vi "Open PNG and convert to 18bit.vi"(8 "error in":errorcluster, 10 "image data":T1={"image type"=0, "image depth"=24, "image"=array[230400 elements], "mask"=[], "colors"=[], "Rectangle"={"left"=0, "top"=0, "right"=320, "bottom"=240}}, 11 "file path (use dialog)":path=path "\\\\vmware-host\\Shared Folders/Downloads/pug.bin") -> (0 "error out":errorcluster, 3 "data":u16[](array[numeric]) format="%.0x")   [LabVIEW 2019]
uses:
  <vilib>/picture/picture.llb/imagedata.ctl
  <userlib>/_OpenG.lib/file/file.llb/File Exists - Scalar__ogtk.vi
panel:
  out "new picture":picture
  out "exists":bool
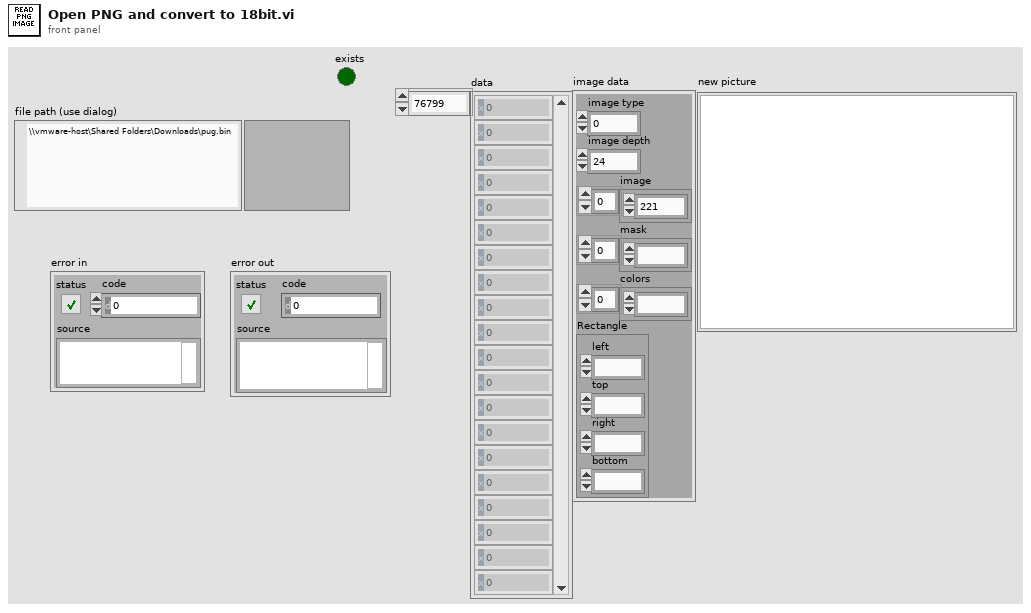
[diagram p1: front panel]
types:
  T1 = typedef "imagedata.ctl" = cluster{"image type":i32, "image depth":i32, "image":u8[], "mask":u8[], "colors":u32[], "Rectangle":cluster{"left":i16, "top":i16, "right":i16, "bottom":i16}}
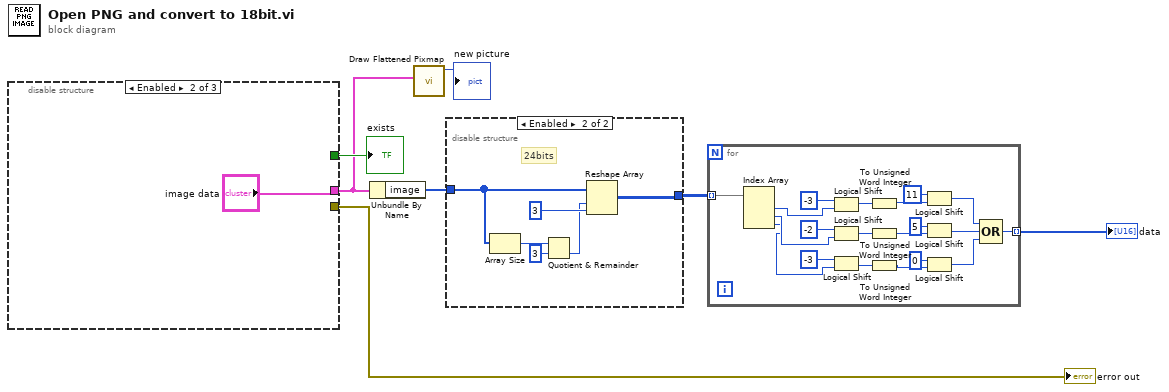
[diagram p0: block diagram]
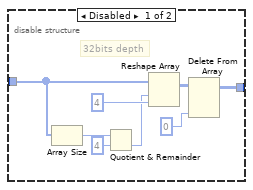
[diagram p2: hidden frame]
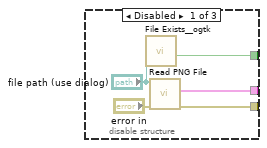
[diagram p3: hidden frame]
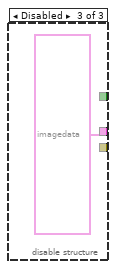
[diagram p4: hidden frame]
diagram:
  n1 = disable-structure shown="Enabled" {
    disable-tunnel: [w11 _ _] -> w4
    disable-tunnel: [w9 _ _] -> w3
    disable-tunnel: [w8 "image data" T1 {"image type"=0, "image depth"=24, "image"=array[230400 elements], "mask"=[], "colors"=[], "Rectangle"={"left"=0, "top"=0, "right"=320, "bottom"=240}} ("image data")] -> w2
    frame Disabled {
      n2 = call-poly <userlib>:"File Exists__ogtk.vi"("file path"="file path (use dialog)") -> ("exists"=w9:bool)  [unwired: 6 in, 1 out]
      n3 = call <vilib>:"Read PNG File.vi"("error in (no error)"="error in", "path to PNG file"="file path (use dialog)") -> ("error out"=w11:errorcluster, "image data"=w8:T1)  [unwired: 7 in, 1 out]
    }
    frame Enabled {
    }
    frame Disabled {
    }
  }
  "error out" <- w4
  "exists" <- w3
  n4 = Unbundle By Name(w2) -> ("image"=w7:u8[])
  n5 = call <vilib>:"Draw Flattened Pixmap.vi"("image data"=w2) -> ("new picture"=→"new picture":picture)  [unwired: 8 in]
  n6 = disable-structure shown="Enabled" {
    disable-tunnel: w7 -> [w16 w24]
    disable-tunnel: [w15 w23] -> w6
    frame Disabled {
      # "32bits depth"
      n7 = Array Size(array=w16) -> (size(s)=w22:i32)
      n8 = Quotient & Remainder(x=w22, y=4) -> (floor(x/y)=w18:i32)  [unwired: 1 out]
      n9 = Reshape Array(w16, w18, 4 ("dimension size")) -> (w20:u8[][])
      n10 = Delete From Array(array=w20, index (col)=0 ("dimension size")) -> (array with subset deleted=w15:u8[][])  [unwired: 2 in, 1 out]
    }
    frame Enabled {
      # "24bits"
      n11 = Array Size(array=w24) -> (size(s)=w28:i32)
      n12 = Quotient & Remainder(x=w28, y=3) -> (floor(x/y)=w25:i32)  [unwired: 1 out]
      n13 = Reshape Array(w24, w25, 3 ("dimension size")) -> (w23:u8[][])
    }
  }
  n14 = for {
    tunnel: w6 -> [w48] mode=indexing
    tunnel: [w32] -> w5 mode=indexing
    n15 = Index Array(array=w48) -> (element #1=w31:u8, element #2=w30:u8, element #3=w29:u8)  [unwired: 3 in]
    n16 = Logical Shift(y=i16 -3, x=w31) -> (x << y=w44:u8)
    n17 = Logical Shift(y=i16 -2, x=w30) -> (x << y=w43:u8)
    n18 = Logical Shift(y=i16 -3, x=w29) -> (x << y=w42:u8)
    n19 = To Unsigned Word Integer(number=w44) -> (unsigned 16bit integer=w41:u16)
    n20 = To Unsigned Word Integer(number=w43) -> (unsigned 16bit integer=w38:u16)
    n21 = To Unsigned Word Integer(number=w42) -> (unsigned 16bit integer=w36:u16)
    n22 = Logical Shift(y=i16 11, x=w41) -> (x << y=w35:u16)
    n23 = Logical Shift(y=i16 5, x=w38) -> (x << y=w34:u16)
    n24 = Logical Shift(y=i16 0, x=w36) -> (x << y=w33:u16)
    n25 = Compound Arithmetic op=OR(w35, w34, w33) -> (w32:u16)
  }
  "data" <- w5
